vi "数据库初始化.vi"(9 "数据库文件名":string, 11 "数据保存路径":path) -> (0 "错误输出":errorcluster, 3 "引用句柄输出":T4)   [LabVIEW 2014]
uses:
  <vilib>/addons/database/Connection.llb/Conn ObjectReference.ctl
  <vilib>/addons/database/Auxilliary.llb/DB Tools Column Info.ctl
  <vilib>/addons/database/Auxilliary.llb/DB Tools DataTypes.ctl
  <vilib>/registry/registry.llb/Registry RtKey.ctl
  <vilib>/registry/registry.llb/Write Registry Value Simple STR.vi
  <vilib>/addons/database/Connection.llb/DB Tools Open Connec (String).vi
  <vilib>/addons/database/NI_Database_API.lvlib
panel:
  out "error out":errorcluster
  in  "column information":T1=[{"column name"="RecordingTime", "data type"=enum."String", "size"=50, "allow null?"=TRUE}, {"column name"="CumulativeOilProduction", "data type"=enum."Double (DBL)", "size"=0, "allow null?"=TRUE}, {"column name"="CumulativeWaterProduction", "data type"=enum."Double (DBL)", "size"=0, "allow null?"=TRUE}, {"column name"="BalanceValue", "data type"=enum."Double (DBL)", "size"=0, "allow null?"=TRUE}, {"column name"="DifferencialPressure", "data type"=enum."Double (DBL)", "size"=0, "allow null?"=TRUE}, {"column name"="Pressure1", "data type"=enum."Double (DBL)", "size"=0, "allow null?"=TRUE}, {"column name"="Pressure2", "data type"=enum."Double (DBL)", "size"=0, "allow null?"=TRUE}, {"column name"="CPPOuterPre", "data type"=enum."Double (DBL)", "size"=0, "allow null?"=TRUE}, {"column name"="CPPTracePre", "data type"=enum."Double (DBL)", "size"=0, "allow null?"=TRUE}, {"column name"="CPPCurrentVol", "data type"=enum."Double (DBL)", "size"=0, "allow null?"=TRUE}, {"column name"="CPPInnerPre", "data type"=enum."Double (DBL)", "size"=0, "allow null?"=TRUE}, {"column name"="FlowSetpointA", "data type"=enum."Double (DBL)", "size"=0, "allow null?"=TRUE}, {"column name"="PressureSetpointA", "data type"=enum."Double (DBL)", "size"=0, "allow null?"=TRUE}, {"column name"="FlowRateA", "data type"=enum."Double (DBL)", "size"=0, "allow null?"=TRUE}, {"column name"="PressuerA", "data type"=enum."Double (DBL)", "size"=0, "allow null?"=TRUE}, {"column name"="FlowSetpointB", "data type"=enum."Double (DBL)", "size"=0, "allow null?"=TRUE}, {"column name"="PressureSetpointB", "data type"=enum."Double (DBL)", "size"=0, "allow null?"=TRUE}, {"column name"="FlowRateB", "data type"=enum."Double (DBL)", "size"=0, "allow null?"=TRUE}, {"column name"="PressuerB", "data type"=enum."Double (DBL)", "size"=0, "allow null?"=TRUE}, {"column name"="InspectionItem", "data type"=enum."String", "size"=0, "allow null?"=TRUE}, {"column name"="WellNumber", "data type"=enum."String", "size"=0, "allow null?"=TRUE}, {"column name"="DateofExperiment", "data type"=enum."String", "size"=0, "allow null?"=TRUE}, {"column name"="NumberofSample", "data type"=enum."String", "size"=0, "allow null?"=TRUE}, {"column name"="LithologicalCharacter ", "data type"=enum."String", "size"=0, "allow null?"=TRUE}, {"column name"="ExperimentalTemperature ", "data type"=enum."String", "size"=0, "allow null?"=TRUE}, {"column name"="SimulatedOilViscosity ", "data type"=enum."String", "size"=0, "allow null?"=TRUE}, {"column name"="InjectionWaterViscosity", "data type"=enum."String", "size"=0, "allow null?"=TRUE}, {"column name"="LengthofRockSample", "data type"=enum."String", "size"=0, "allow null?"=TRUE}, {"column name"="PoreVolume ", "data type"=enum."String", "size"=0, "allow null?"=TRUE}, {"column name"="CoreDepth ", "data type"=enum."String", "size"=0, "allow null?"=TRUE}, {"column name"="AirPermeability ", "data type"=enum."String", "size"=0, "allow null?"=TRUE}, {"column name"="SimulatedOilDensity", "data type"=enum."String", "size"=0, "allow null?"=TRUE}, {"column name"="InjectionWaterDensity", "data type"=enum."String", "size"=0, "allow null?"=TRUE}, {"column name"="RockSampleDiameter ", "data type"=enum."String", "size"=0, "allow null?"=TRUE}, {"column name"="Porosity", "data type"=enum."String", "size"=0, "allow null?"=TRUE}, {"column name"="InletPressure", "data type"=enum."String", "size"=0, "allow null?"=TRUE}, {"column name"="OutletPressure", "data type"=enum."String", "size"=0, "allow null?"=TRUE}, {"column name"="IrreducibleWaterSaturation", "data type"=enum."String", "size"=0, "allow null?"=TRUE}, {"column name"="SectionalArea", "data type"=enum."String", "size"=0, "allow null?"=TRUE}, {"column name"="VolumeOfRockSample", "data type"=enum."String", "size"=0, "allow null?"=TRUE}]
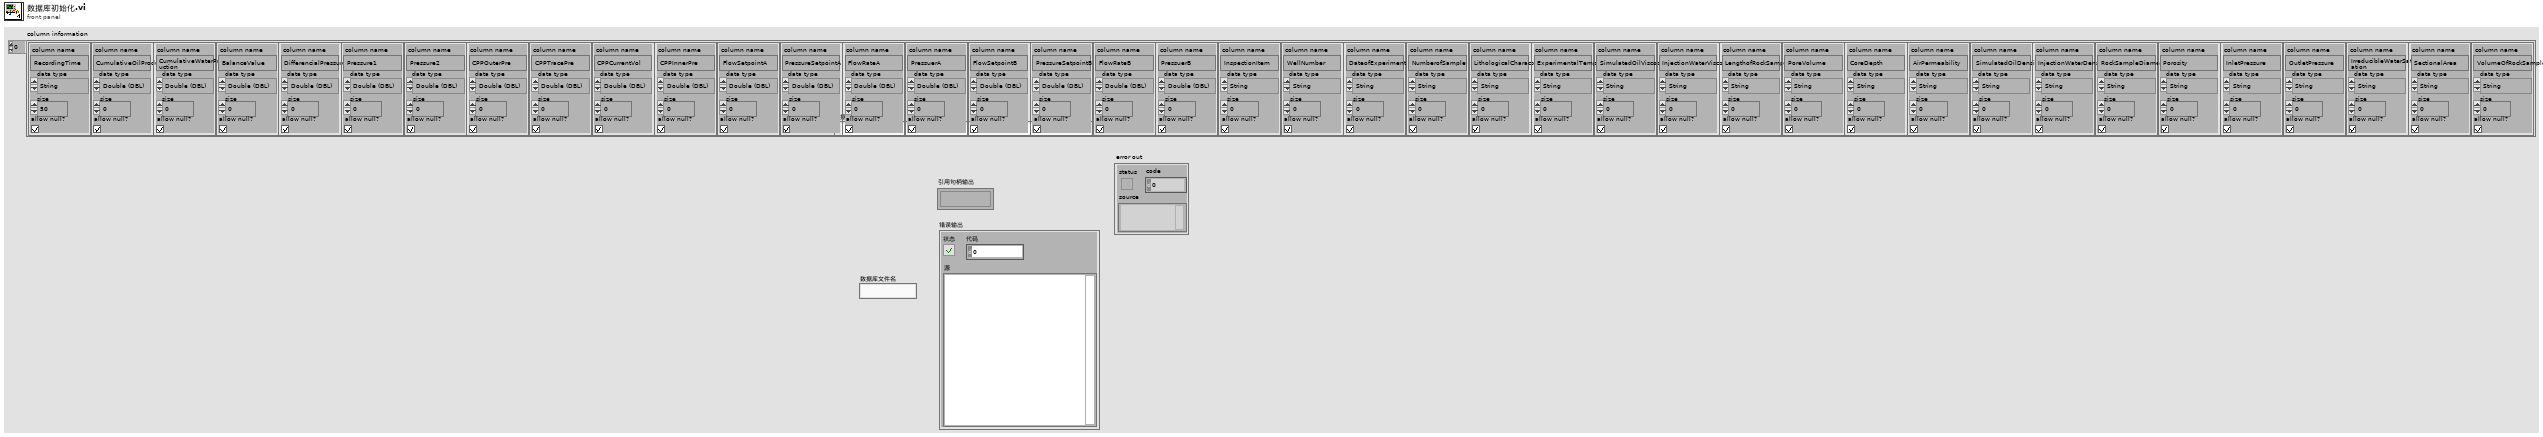
[diagram p1: front panel]
types:
  T1 = typedef "控件 1.ctl" = T2[]
  T2 = typedef "NI_Database_API.lvlib/DB Tools Column Info.ctl" = cluster{"column name":string, "data type":T3, "size":i32, "allow null?":bool}
  T3 = typedef "NI_Database_API.lvlib/DB Tools DataTypes.ctl" = enum16{"String", "Long (I32)", "Single (SGL)", "Double (DBL)", "Date/Time", "Binary"}
  T4 = typedef "NI_Database_API.lvlib/Conn ObjectReference.ctl" = refnum<k1>
  T5 = typedef "Registry RtKey.ctl" = enum32{"HKEY_CLASSES_ROOT", "HKEY_CURRENT_USER", "HKEY_LOCAL_MACHINE", "HKEY_USERS", "HKEY_PERFORMANCE_DATA", "HKEY_CURRENT_CONFIG", "HKEY_DYN_DATA"}
  T6 = typedef "Registry refnum.ctl" = refnum<k1>
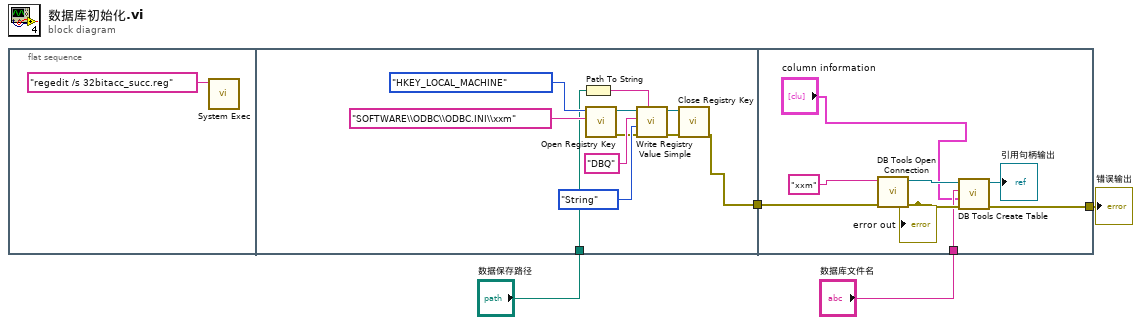
[diagram p0: block diagram]
diagram:
  n1 = flat-sequence {
    tunnel: "数据保存路径" -> [w9]
    tunnel: [w7] -> w1
    tunnel: [w20] -> w4
    tunnel: "数据库文件名" -> [w21]
    tunnel: w1 -> [w17]
    frame #0 {
      n2 = call <vilib>:"System Exec.vi"("command line"="regedit /s 32bitacc_succ.reg") -> ()  [unwired: 7 in, 4 out]
    }
    frame #1 {
      n3 = Path To String(path=w9) -> (string=w14:string)
      n4 = call <vilib>:"Open Registry Key.vi"("subkey"="SOFTWARE\\ODBC\\ODBC.INI\\xxm", "root key (HKEY_LOCAL_MACHINE)"=Registry_RtKey."HKEY_LOCAL_MACHINE") -> ("error out"=w6:errorcluster, "refnum out"=w11:T6)  [unwired: 8 in]
      n5 = call-poly <vilib>:"Write Registry Value Simple.vi"("String/Binary data"=w14, "error in (no error)"=w6, "simple data type"=enum16{"String", "Binary", "DWORD"}."String", "value"="DBQ", "refnum"=w11) -> ("error out"=w8:errorcluster, "refnum out"=w16:T6)  [unwired: 3 in]
      n6 = call <vilib>:"Close Registry Key.vi"("error in (no error)"=w8, "refnum"=w16) -> ("error out"=w7:errorcluster)  [unwired: 5 in]
    }
    frame #2 {
      n7 = call-poly <vilib>:"DB Tools Open Connection.vi"("error in (no error)"=w17, "connection information"="xxm" ("value")) -> ("error out"=w23:errorcluster, "connection reference"=w24:T4)  [unwired: 6 in]
      "error out" <- w23
      n8 = call <vilib>:"DB Tools Create Table.vi"("error in (no error)"=w23, "column information"="column information", "table"=w21, "connection reference"=w24) -> ("error out"=w20:errorcluster, "connection reference out"=→"引用句柄输出":T4)  [unwired: 4 in]
    }
  }
  "错误输出" <- w4
